vi "Get SLSC Module By Name.vi"(8 "error in (no error)":errorcluster, 10 "Name":string, 11 "SLSC Chassis":u64) -> (0 "error out":errorcluster, 1 "Found":bool, 2 "SLSC Module":u64, 3 "SLSC Chassis out":u64)   [LabVIEW 2020, in "VeriStand SLSC Scripting.lvlib"]
uses:
  VeriStand SLSC Scripting.lvlib
  NationalInstruments.VeriStand.SystemDefinitionAPI
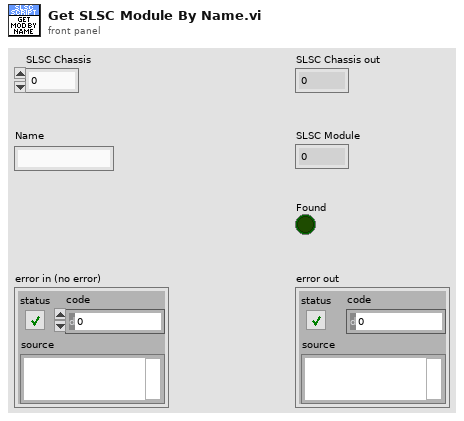
[diagram p1: front panel]
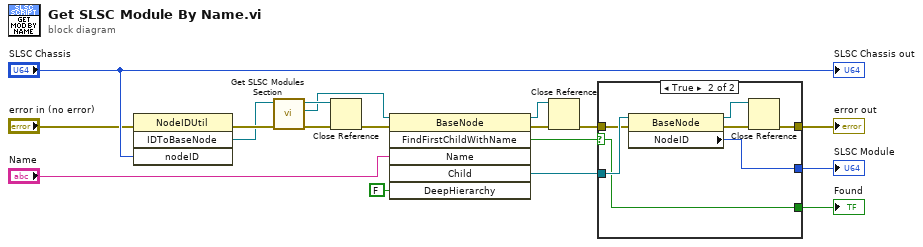
[diagram p0: block diagram]
diagram:
  n1 = invoke class="NodeIDUtil" method="IDToBaseNode"(error in="error in (no error)", "nodeID"="SLSC Chassis") -> (error out=w6:errorcluster, "IDToBaseNode"=w5:refnum<k24>)  [unwired: 2 in, 2 out]
  n2 = call "Get SLSC Modules Section.vi"("error in (no error)"=w6, "SLSC Chassis"=w5) -> ("error out"=w4:errorcluster, "Modules Section"=w1:refnum<k24>, "SLSC Chassis out"=w3:refnum<k24>)  [unwired: 7 in]
  n3 = Close Reference(reference=w3, error in (no error)=w4) -> (error out=w2:errorcluster)
  n4 = invoke class="BaseNode" method="FindFirstChildWithName"(reference=w1, error in=w2, "Name"="Name", "DeepHierarchy"=FALSE) -> (reference out=w10:refnum<k24>, error out=w13:errorcluster, "FindFirstChildWithName"=w9:bool, "Child"=w12:refnum<k24>)  [unwired: 2 in, 2 out]
  n5 = Close Reference(reference=w10, error in (no error)=w13) -> (error out=w11:errorcluster)
  n6 = case shown="True" w9 {
    selector: w9 -> [w19 w24]
    tunnel: [w20 w22] -> w7
    tunnel: [_ w27] -> w16
    tunnel: w12 -> [_ w26]
    tunnel: w11 -> [w20 w25]
    tunnel: [w19 w24] -> w8
    frame False {
    }
    frame True {
      n7 = property class="BaseNode"(reference=w26, error in=w25) -> (reference out=w21:refnum<k24>, error out=w23:errorcluster, "NodeID"=w27:u64)
      n8 = Close Reference(reference=w21, error in (no error)=w23) -> (error out=w22:errorcluster)
    }
  }
  "error out" <- w7
  "SLSC Module" <- w16
  "Found" <- w8
  "SLSC Chassis out" <- "SLSC Chassis"
